vi "find_1f2f_diag.vi"(9 "FFT - (RMS)":cluster{"f0":dbl, "df":dbl, "magnitude":dbl[]}, 10 "Peak FWHM":dbl, 11 "Central Frequency":dbl) -> (1 "Cluster":cluster{dbl, dbl, dbl, dbl}, 2 "2f Frequency":dbl[](array[numeric])=[6.0], 3 "2f Peak Amplitude (mVrms/Vdc)":dbl=0.004981012167818904, 4 "1f Peak Amplitude(mVrms/Vdc)":dbl, 5 "1f Frequency":dbl[](array[numeric]))   [LabVIEW 2015]
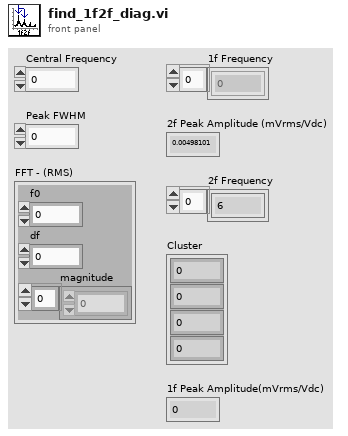
[diagram p1: front panel]
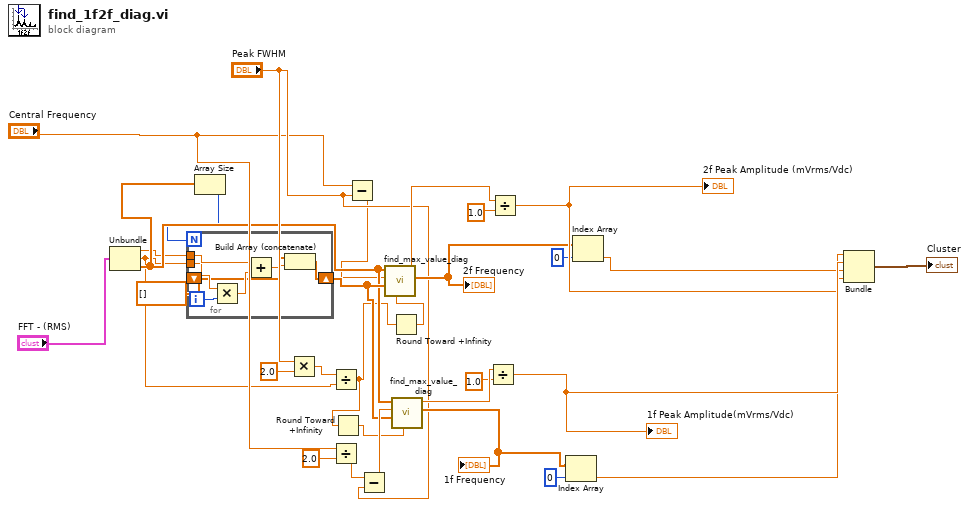
[diagram p0: block diagram]
diagram:
  n1 = Unbundle("FFT - (RMS)") -> ("f0"=w8:dbl, "df"=w11:dbl, "magnitude"=w12:dbl[])
  n2 = Array Size(array=w12) -> (size(s)=w7:i32)
  n3 = for {
    N: w7 -> [_]
    tunnel: w8 -> [w38]
    tunnel: w11 -> [w35]
    shift-right: [w33] -> w13
    shift-left: dbl[] [] -> [w32]
    i -> [w37]
    n4 = Multiply(x=w35, y=w37) -> (x*y=w36:dbl)
    n5 = Add(x=w38, y=w36) -> (x+y=w34:dbl)
    n6 = Build Array (concatenate)(w32, w34) -> (w33:dbl[])
  }
  n7 = Multiply(x="Peak FWHM", y=2.0) -> (x*y=w10:dbl)
  n8 = Divide(x=w10, y=w11) -> (x/y=w2:dbl)
  n9 = Divide(x="Central Frequency", y=2.0) -> (x/y=w16:dbl)
  n10 = Round Toward +Infinity(x=w2) -> (ceil(x): smallest int >= x=w3:dbl)
  n11 = Subtract(x="Central Frequency", y="Peak FWHM") -> (x-y=w5:dbl)
  n12 = Subtract(x=w16, y="Peak FWHM") -> (x-y=w18:dbl)
  n13 = Round Toward +Infinity(x=w2) -> (ceil(x): smallest int >= x=w1:dbl)
  n14 = call "find_max_value_diag.vi"("length"=w1, "Frequency array"=w13, "Lower Freq"=w5, "Amplitude Array"=w12) -> ("Frequency"=w21:dbl[], "Peak Amplitude"=w27:dbl)  [unwired: 6 in]
  "2f Frequency" <- w21
  n15 = call "find_max_value_diag.vi"("length"=w3, "Frequency array"=w13, "Lower Freq"=w18, "Amplitude Array"=w12) -> ("Frequency"=w19:dbl[], "Peak Amplitude"=w30:dbl)  [unwired: 6 in]
  "1f Frequency" <- w19
  n16 = Divide(x=w30, y=1.0) -> (x/y=w31:dbl)
  "1f Peak Amplitude(mVrms/Vdc)" <- w31
  n17 = Divide(x=w27, y=1.0) -> (x/y=w28:dbl)
  "2f Peak Amplitude (mVrms/Vdc)" <- w28
  n18 = Index Array(array=w19, index=0) -> (element=w23:dbl)
  n19 = Index Array(array=w21, index=0) -> (element=w24:dbl)
  n20 = Bundle(w23, w31, w24, w28) -> (→"Cluster":cluster{dbl, dbl, dbl, dbl})  [unwired: 1 in]
